vi "SPIE Decide.vi"(6 "Previous Radius":dbl, 7 "Compass Bearing_k":dbl, 9 "Threshold":u32, 10 "SICK Data":u32[](array[numeric]), 11 "Decide Bearing_(k+1)":dbl) -> (1 "Turning Radius":dbl, 2 "Speed":dbl, 3 "Decide Bearing_k":dbl, 4 "error":dbl)   [LabVIEW 2009]
uses:
  Valley.ctl
panel:
  out "Array":T1[](array[typedef])
  out "decided heading":i32
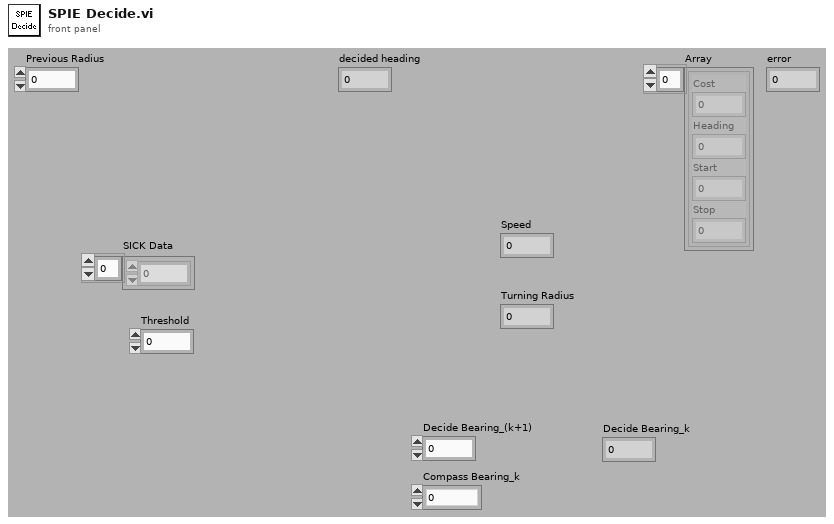
[diagram p1: front panel]
types:
  T1 = typedef "Valley.ctl" = cluster{"Cost":dbl, "Heading":i32, "Start":i32, "Stop":i32}
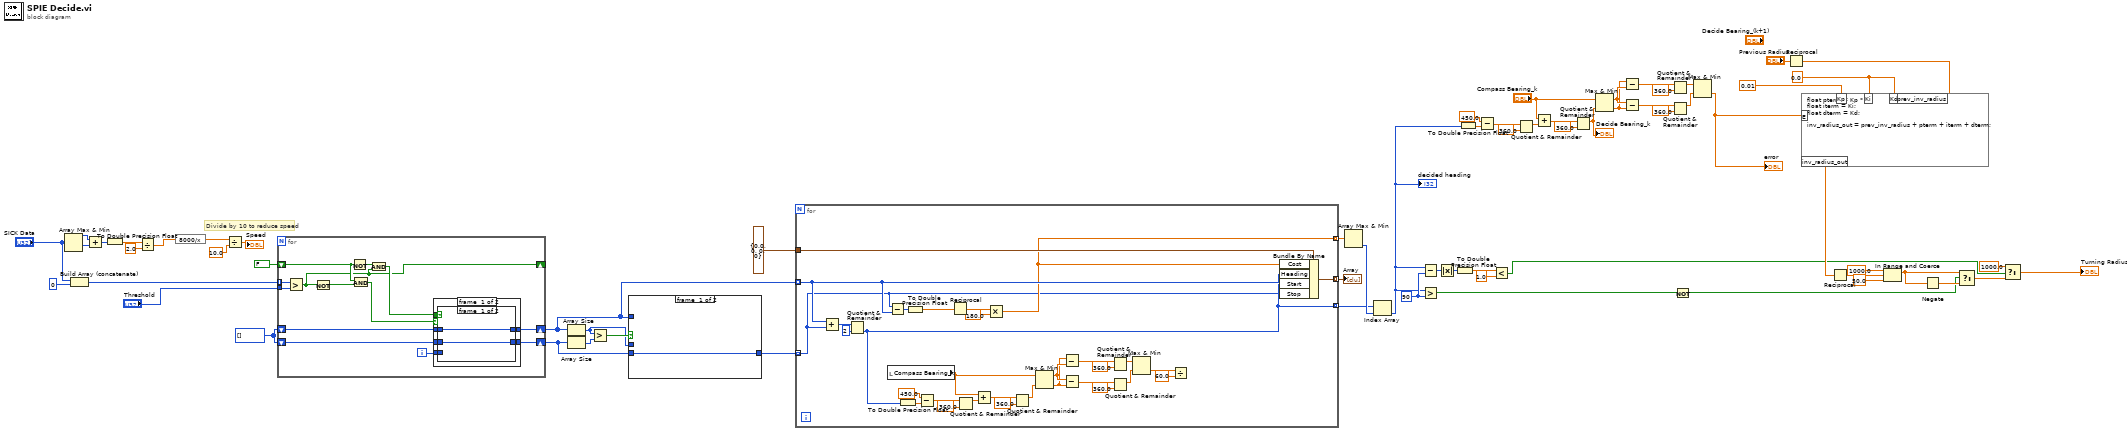
[diagram p0: block diagram]
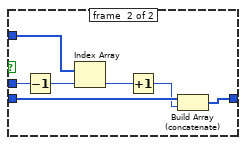
[diagram p2: hidden frame]
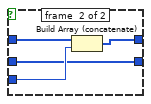
[diagram p3: hidden frame]
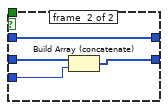
[diagram p4: hidden frame]
diagram:
  w28 = 0.0 ("input variable")
  w57 = i32[] [] ("SICK Data 2")
  w43 = 90 ("y")
  # "Divide by 10 to reduce speed"
  n1 = Array Max & Min(array="SICK Data") -> (max value=w66:u32, min value=w65:u32)  [unwired: 2 out]
  n2 = Build Array (concatenate)("SICK Data", u32 0 ("Numeric")) -> (w39:u32[])
  n3 = Add(x=w66, y=w65) -> (x+y=w64:u32)
  n4 = To Double Precision Float(number=w64) -> (double precision float=w62:dbl)
  n5 = Divide(x=w62, y=2.0) -> (x/y=w60:dbl)
  n6 = expression code="8000/x"(w60) -> (w3:dbl)
  n7 = Divide(x=w3, y=10.0) -> (x/y=→"Speed":dbl)
  n8 = for {
    tunnel: w39 -> [w79] mode=indexing
    shift-right: [w68] -> _
    shift-left: FALSE -> [w76]
    tunnel: "Threshold" -> [w78]
    shift-right: [w71] -> w51
    shift-left: w57 -> [w73]
    shift-right: [w69] -> w54
    shift-left: w57 -> [w72]
    i -> [w70]
    n9 = Greater?(x=w79, y=w78) -> (0:w68:bool)
    n10 = Not(x=w68) -> (.not. x?=w77:bool)
    n11 = Not(x=w76) -> (.not. x?=w75:bool)
    n12 = And(x=w76, y=w77) -> (x .and. y?=w67:bool)
    n13 = And(x=w75, y=w68) -> (x .and. y?=w74:bool)
    n14 = case shown="True" w67 {
      tunnel: w74 -> [w85 _]
      tunnel: w73 -> [w84 w92]
      tunnel: w72 -> [w83 w94]
      tunnel: [w82 w92] -> w71
      tunnel: w70 -> [w81 w95]
      tunnel: [w80 w93] -> w69
      frame #0 {
        n15 = case shown="False" w85 {
          tunnel: w84 -> [w87 w91]
          tunnel: w83 -> [w86 w88]
          tunnel: [w87 w90] -> w82
          tunnel: w81 -> [_ w89]
          tunnel: [w86 w88] -> w80
          frame #0 {
          }
          frame #1 {
            n16 = Build Array (concatenate)(w91, w89) -> (w90:i32[])
          }
        }
      }
      frame #1 {
        n17 = Build Array (concatenate)(w94, w95) -> (w93:i32[])
      }
    }
  }
  n18 = Array Size(array=w51) -> (size(s)=w53:i32)
  n19 = Array Size(array=w54) -> (size(s)=w56:i32)
  n20 = Greater?(x=w53, y=w56) -> (0:w55:bool)
  n21 = case shown="True" w55 {
    tunnel: w54 -> [w96 w103]
    tunnel: w51 -> [_ w102]
    tunnel: w53 -> [_ w100]
    tunnel: [w96 w97] -> w52
    frame #0 {
    }
    frame #1 {
      n22 = Decrement(x=w100) -> (x-1=w101:i32)
      n23 = Index Array(array=w102, index=w101) -> (element=w99:i32)
      n24 = Increment(x=w99) -> (x+1=w98:i32)
      n25 = Build Array (concatenate)(w103, w98) -> (w97:i32[])
    }
  }
  n26 = for {
    tunnel: w52 -> [w104] mode=indexing
    tunnel: w51 -> [w130] mode=indexing
    tunnel: T1 {"Cost"=0.0, "Heading"=0, "Start"=0, "Stop"=0} ("Cluster") -> [w134]
    tunnel: [w131] -> w46 mode=indexing
    tunnel: [w106] -> w49 mode=indexing
    tunnel: [w112] -> w47 mode=indexing
    n27 = Add(x=w130, y=w104) -> (x+y=w133:i32)
    n28 = Quotient & Remainder(x=w133, y=2) -> (floor(x/y)=w112:i32)  [unwired: 1 out]
    n29 = local read "Compass Bearing_k"() -> (w129:dbl)
    n30 = Subtract(x=w104, y=w130) -> (x-y=w109:i32)
    n31 = To Double Precision Float(number=w112) -> (double precision float=w125:dbl)
    n32 = To Double Precision Float(number=w109) -> (double precision float=w108:dbl)
    n33 = Subtract(x=450.0, y=w125) -> (x-y=w127:dbl)
    n34 = Reciprocal(x=w108) -> (1/x=w107:dbl)
    n35 = Quotient & Remainder(x=w127, y=360.0) -> (x-y*floor(x/y)=w122:dbl)  [unwired: 1 out]
    n36 = Add(x=w129, y=w122) -> (x+y=w123:dbl)
    n37 = Multiply(x=w107, y=180.0) -> (x*y=w106:dbl)
    n38 = Quotient & Remainder(x=w123, y=360.0) -> (x-y*floor(x/y)=w113:dbl)  [unwired: 1 out]
    n39 = Max & Min(x=w129, y=w113) -> (max(x,y)=w119:dbl, min(x,y)=w118:dbl)
    n40 = Subtract(x=w118, y=w119) -> (x-y=w121:dbl)
    n41 = Subtract(x=w119, y=w118) -> (x-y=w116:dbl)
    n42 = Quotient & Remainder(x=w121, y=360.0) -> (x-y*floor(x/y)=w115:dbl)  [unwired: 1 out]
    n43 = Quotient & Remainder(x=w116, y=360.0) -> (x-y*floor(x/y)=w114:dbl)  [unwired: 1 out]
    n44 = Max & Min(x=w115, y=w114) -> (min(x,y)=w111:dbl)  [unwired: 1 out]
    n45 = Divide(x=w111, y=60.0) -> ()  [unwired: 1 out]
    n46 = Bundle By Name(cluster=w134, "Cost"=w106, "Heading"=w112, "Start"=w130, "Stop"=w104) -> (w131:T1)
  }
  "Array" <- w46
  n47 = Array Max & Min(array=w49) -> (min index (indices)=w48:i32)  [unwired: 3 out]
  n48 = Index Array(array=w47, index=w48) -> (element=w34:i32)
  "decided heading" <- w34
  n49 = Subtract(x=w34, y=w43) -> (x-y=w42:i32)
  n50 = Greater?(x=w34, y=w43) -> (0:w61:bool)
  n51 = Absolute Value(x=w42) -> (abs(x)=w41:i32)
  n52 = To Double Precision Float(number=w41) -> (double precision float=w40:dbl)
  n53 = To Double Precision Float(number=w34) -> (double precision float=w33:dbl)
  n54 = Subtract(x=450.0, y=w33) -> (x-y=w36:dbl)
  n55 = Less?(x=w40, y=1.0) -> (x < y?=w23:bool)
  n56 = Quotient & Remainder(x=w36, y=360.0) -> (x-y*floor(x/y)=w30:dbl)  [unwired: 1 out]
  n57 = Add(x="Compass Bearing_k", y=w30) -> (x+y=w31:dbl)
  n58 = Quotient & Remainder(x=w31, y=360.0) -> (x-y*floor(x/y)=w12:dbl)  [unwired: 1 out]
  "Decide Bearing_k" <- w12
  n59 = Max & Min(x="Compass Bearing_k", y=w12) -> (max(x,y)=w19:dbl, min(x,y)=w18:dbl)
  n60 = Subtract(x=w18, y=w19) -> (x-y=w21:dbl)
  n61 = Subtract(x=w19, y=w18) -> (x-y=w16:dbl)
  n62 = Quotient & Remainder(x=w21, y=360.0) -> (x-y*floor(x/y)=w15:dbl)  [unwired: 1 out]
  n63 = Quotient & Remainder(x=w16, y=360.0) -> (x-y*floor(x/y)=w14:dbl)  [unwired: 1 out]
  n64 = Not(x=w61) -> (.not. x?=w4:bool)
  n65 = Max & Min(x=w15, y=w14) -> (min(x,y)=w11:dbl)  [unwired: 1 out]
  "error" <- w11
  n66 = Reciprocal(x="Previous Radius") -> (1/x=w22:dbl)
  n67 = formula code="float pterm = Kp * E;\nfloat iterm = Ki;\nfloat dterm = Kd;\n\ninv_radius_out = prev_inv_radius + pterm + iterm + dterm;"("E"=w11, "Kp"=0.01 ("input variable"), "Ki"=w28, "Kd"=w28, "prev_inv_radius"=w22) -> ("inv_radius_out"=w24:dbl)
  n68 = Reciprocal(x=w24) -> (1/x=w7:dbl)
  n69 = In Range and Coerce(upper limit=1000.0, x=w7, lower limit=50.0) -> (coerced(x)=w6:dbl)  [unwired: 1 out]
  n70 = Negate(x=w6) -> (-x=w25:dbl)
  n71 = Select(t=w6, s=w4, f=w25) -> (s? t:f=w26:dbl)
  n72 = Select(t=1000.0 ("f"), s=w23, f=w26) -> (s? t:f=→"Turning Radius":dbl)
